vi "MetaClientPreProc.vi"(8 "error in (no error)":errorcluster, 11 "File Paths":T1={"Local Save Path"=path "\\\\smbhome.uscs.susx.ac.uk\\cv222/Desktop/data", "Newton Save Path"=path "Z:/#Projects/Entanglement/data", "File Name"="test", "LocalSave"=TRUE}) -> (0 "error out":errorcluster, 3 "steps":i32, 4 "Stop?":bool=TRUE)   [LabVIEW 2019]
uses:
  controls/FilePaths.ctl
  controls/GlobalExp.vi
  Global.lvlib
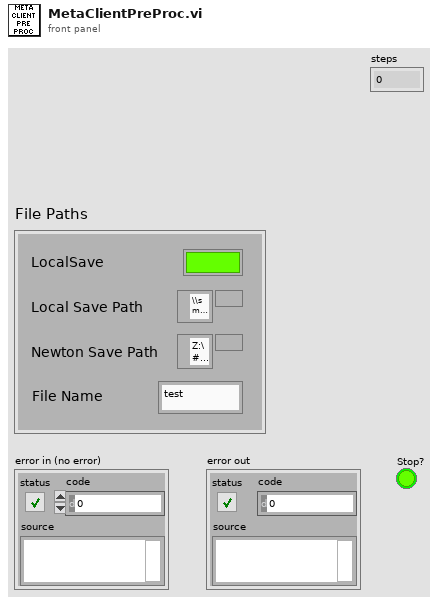
[diagram p1: front panel]
types:
  T1 = typedef "FilePaths.ctl" = cluster{"Local Save Path":path, "Newton Save Path":path, "File Name":string, "LocalSave":bool}
  T2 = enum16{"Standard", "Buffered", "CRLF", "Immediate"}
  T3 = typedef "MasterExpControl.ctl" = cluster{"Main Steps":dbl, "Main Runs":dbl, "ExpStatus":enum16{"Innit", "Stop", "Idle", "MainRunning", "AuxRunning"}, "Main Current Step":dbl, "ExpNum":dbl, "NewData":bool, "date":string, "command":string, "Stop":bool, "Pause":bool, "Mathematica":string, "Main/Meta":bool, "UpdateMath":bool, "Camera":bool, "MetaExpOver":bool, "NextMetaExp":bool}
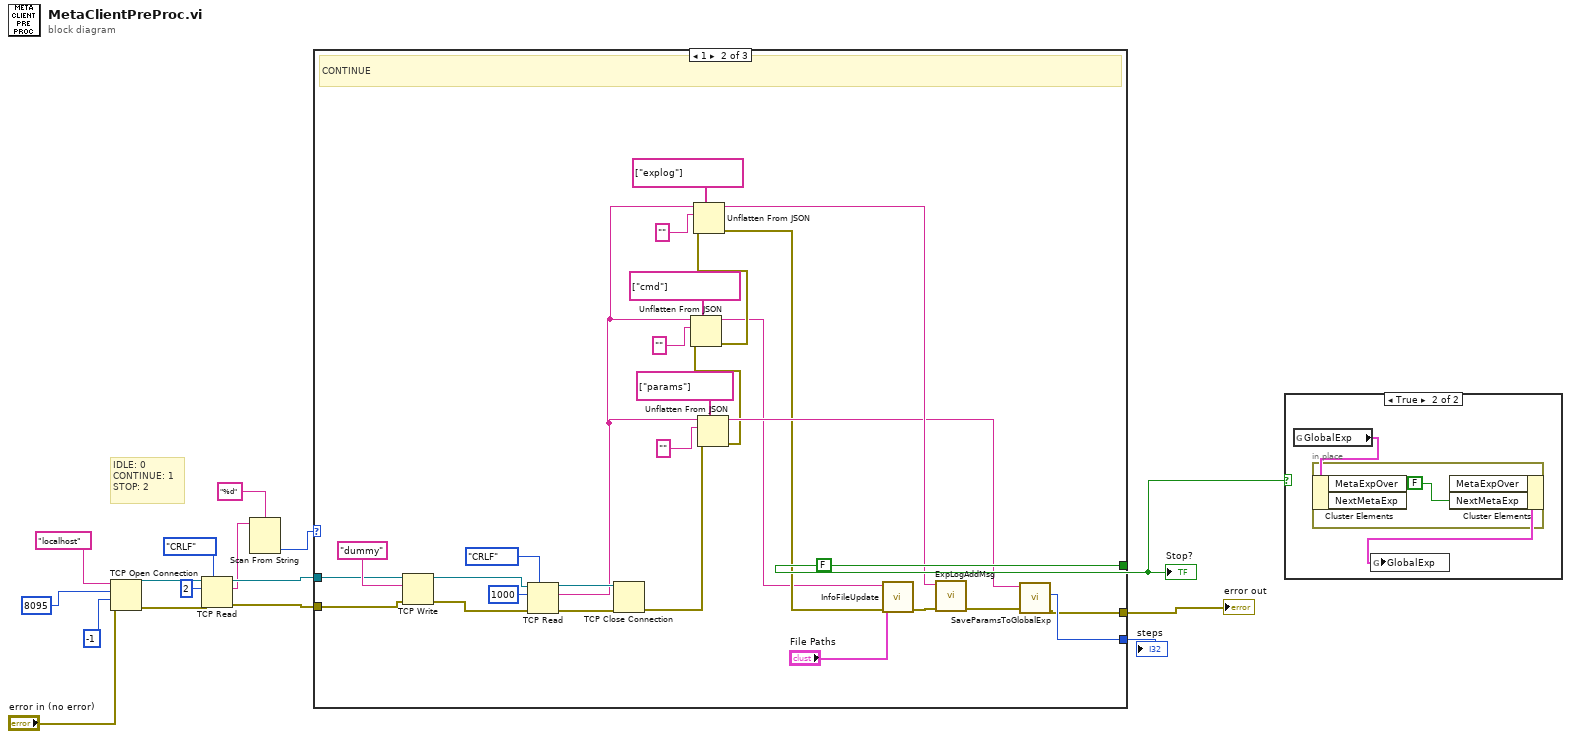
[diagram p0: block diagram]
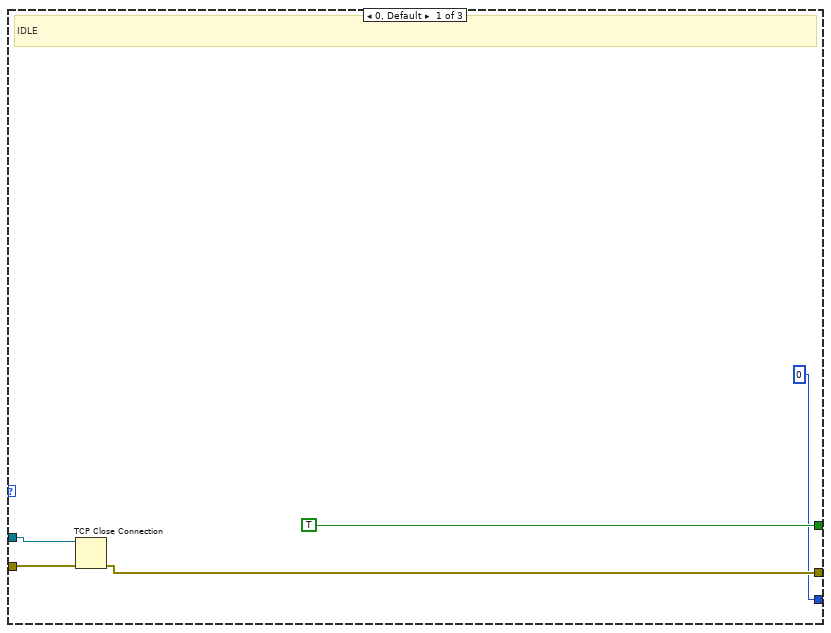
[diagram p3: hidden frame]
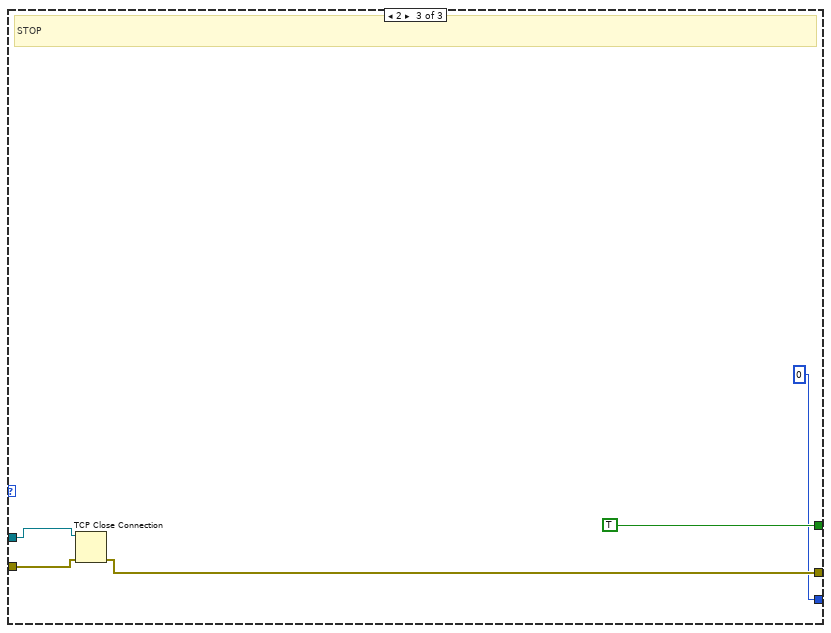
[diagram p4: hidden frame]
diagram:
  # "IDLE: 0\nCONTINUE: 1\nSTOP: 2"
  n1 = TCP Open Connection(address="localhost", remote port or service name=u16 8095, timeout ms (60000)=-1, error in (no error)="error in (no error)") -> (connection ID=w10:refnum<k5>, error out=w9:errorcluster)  [unwired: 1 in]
  n2 = TCP Read(connection ID=w10, bytes to read=2, error in (no error)=w9, 7:T2."CRLF" ("mode (standard)")) -> (connection ID out=w12:refnum<k5>, data out=w5:string, error out=w11:errorcluster)  [unwired: 1 in]
  n3 = Scan From String(format string="%d", input string=w5) -> (output 1=w3:i32)  [unwired: 3 in, 3 out]
  n4 = case shown="1" w3 {
    tunnel: w12 -> [w20 w46 w55]
    tunnel: w11 -> [w21 w43 w54]
    tunnel: [TRUE FALSE TRUE] -> w1
    tunnel: [w18 w22 w52] -> w6
    tunnel: [0 w30 0] -> w2
    frame 0, Default {
      # "IDLE"
      n5 = TCP Close Connection(connection ID=w20, error in (no error)=w21) -> (error out=w18:errorcluster)  [unwired: 1 in, 1 out]
    }
    frame 1 {
      # "CONTINUE"
      n6 = TCP Write(connection ID=w46, data in="dummy", error in (no error)=w43) -> (connection ID out=w45:refnum<k5>, error out=w44:errorcluster)  [unwired: 1 in, 1 out]
      n7 = TCP Read(connection ID=w45, bytes to read=1000, error in (no error)=w44, 7:T2."CRLF" ("mode (standard)")) -> (connection ID out=w41:refnum<k5>, data out=w34:string, error out=w42:errorcluster)  [unwired: 1 in]
      n8 = TCP Close Connection(connection ID=w41, error in (no error)=w42) -> (error out=w27:errorcluster)  [unwired: 1 in, 1 out]
      n9 = Unflatten From JSON(path=string[] ["params"], JSON string=w34, type and defaults="", error in (no error)=w27) -> (value=w29:string, error out=w26:errorcluster)  [unwired: 3 in]
      n10 = Unflatten From JSON(path=string[] ["cmd"], JSON string=w34, type and defaults="", error in (no error)=w26) -> (value=w23:string, error out=w25:errorcluster)  [unwired: 3 in]
      n11 = Unflatten From JSON(path=string[] ["explog"], JSON string=w34, type and defaults="", error in (no error)=w25) -> (value=w33:string, error out=w24:errorcluster)  [unwired: 3 in]
      n12 = call "InfoFileUpdate.vi"("error in"=w24, "File Paths"="File Paths", "info msg"=w23) -> ("error out"=w32:errorcluster)  [unwired: 8 in]
      n13 = call "ExpLogAddMsg.vi"("error in (no error)"=w32, "msg in"=w33) -> ("error out"=w31:errorcluster)  [unwired: 9 in]
      n14 = call "SaveParamsToGlobalExp.vi"("error in"=w31, "FlattendJSon in"=w29) -> ("error out"=w22:errorcluster, "steps"=w30:i32)  [unwired: 7 in, 1 out]
    }
    frame 2 {
      # "STOP"
      n15 = TCP Close Connection(connection ID=w55, error in (no error)=w54) -> (error out=w52:errorcluster)  [unwired: 1 in, 1 out]
    }
  }
  "Stop?" <- w1
  "error out" <- w6
  "steps" <- w2
  n16 = case shown="True" w1 {
    frame False {
    }
    frame True {
      n17 = global read "GlobalExp.vi" "GlobalExp"() -> (w56:T3)
      n18 = in-place {
        w58 = FALSE ("MetaExpOver")
        n19 = in-place-cluster #1(w56) -> ()  [unwired: 2 out]
        n20 = in-place-cluster #1("MetaExpOver"=w58, "NextMetaExp"=w58) -> (w57:T3)
      }
      n21 = global write "GlobalExp.vi" "GlobalExp"(w57) -> ()
    }
  }
